vi "Setting Max Current e Modalita.vi"(0 "VISA resource name":refnum<visa-resource-name>, 5 "error in (no error)":errorcluster) -> (6 "VISA resource name out":refnum<visa-resource-name>, 8 "error out":errorcluster)   [LabVIEW 2018]
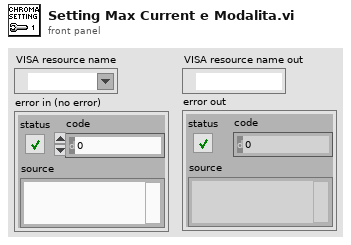
[diagram p1: front panel]
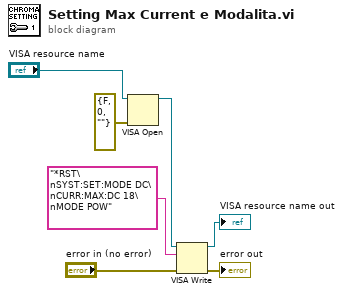
[diagram p0: block diagram]
diagram:
  n1 = VISA Open(error in (no error)=errorcluster {"status"=FALSE, "code"=0, "source"=""}, VISA resource name="VISA resource name") -> (VISA resource name=w1:refnum<visa-resource-name>)  [unwired: 3 in, 1 out]
  n2 = VISA Write(VISA resource name=w1, write buffer="*RST\nSYST:SET:MODE DC\nCURR:MAX:DC 18\nMODE POW", error in (no error)="error in (no error)") -> (VISA resource name out=→"VISA resource name out":refnum<visa-resource-name>, error out=→"error out":errorcluster)  [unwired: 1 out]
